vi "Read Resource Descriptor.vi"(8 "error in (no error)":errorcluster, 11 "SG Path in":refnum<class "SG Path.lvclass">) -> (0 "error out":errorcluster, 2 "Resource Descriptor":string, 3 "SG Path out":refnum<class "SG Path.lvclass">)   [LabVIEW 2023, in "RFFixtureCharact.Public.lvlib" / "SG Path.lvclass"]
uses:
  SG Path.lvclass
  SG Path.lvclass/SG Path.ctl
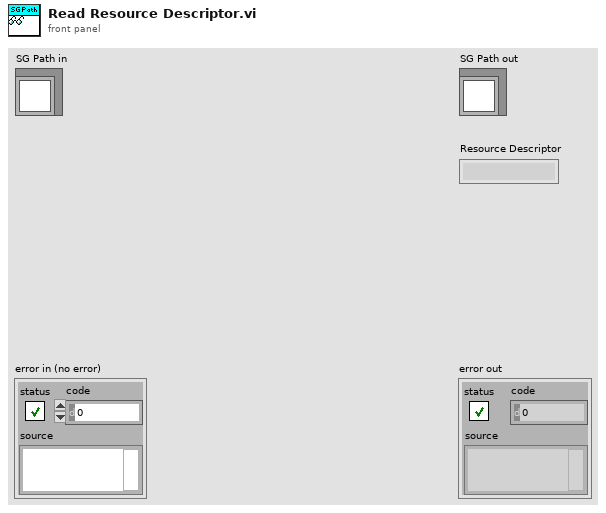
[diagram p1: front panel]
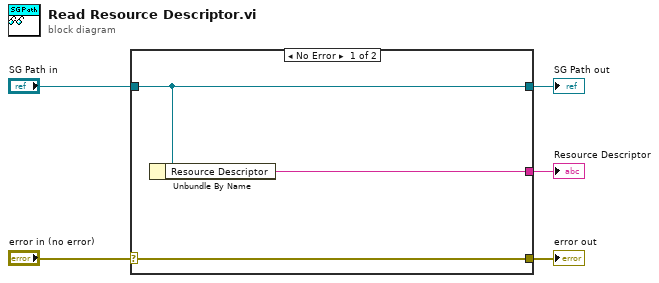
[diagram p0: block diagram]
diagram:
  n1 = case shown="No Error" "error in (no error)" {
    selector: "error in (no error)" -> [w8 w9]
    tunnel: [w8 w9] -> w4
    tunnel: [w7 w10] -> w2
    tunnel: "SG Path in" -> [w7 w10]
    tunnel: [w6 _] -> w1
    frame No Error {
      n2 = Unbundle By Name(w7) -> ("Resource Descriptor"=w6:string)
    }
    frame Error {
    }
  }
  "error out" <- w4
  "SG Path out" <- w2
  "Resource Descriptor" <- w1
